vi "Main.vi"() -> ()   [LabVIEW 2013]
panel:
  in  "Continue":bool
  in  "Team Number":string
  in  "Other Name":string
  in  "Name":string(combo)="Other"
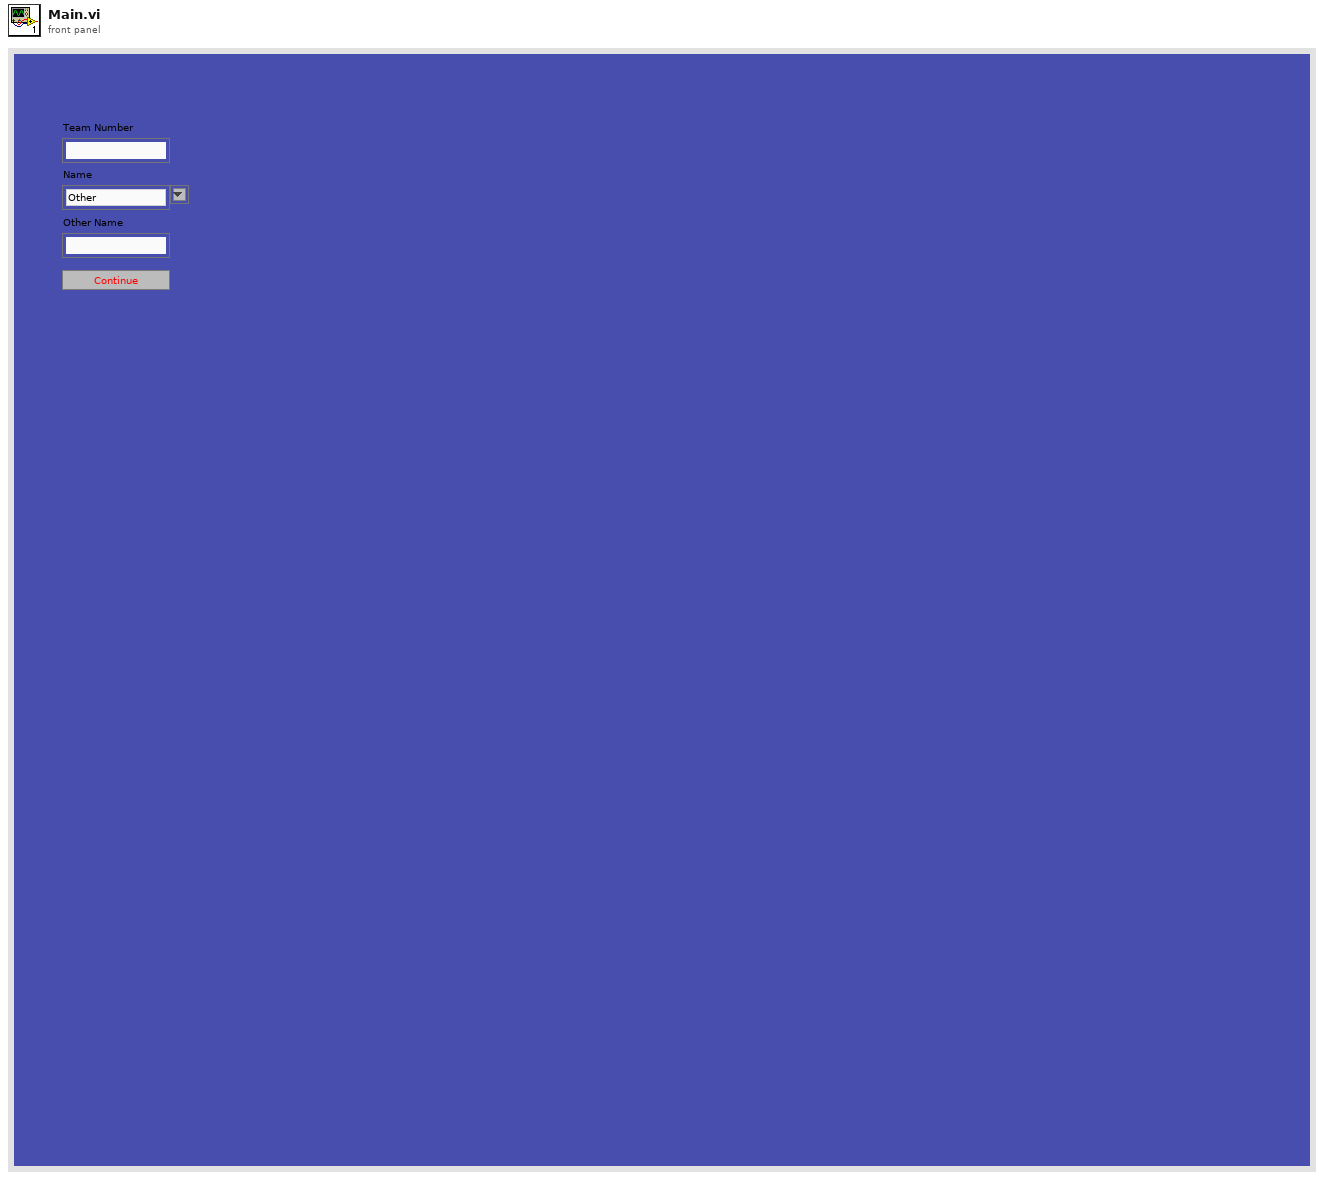
[diagram p1: front panel]
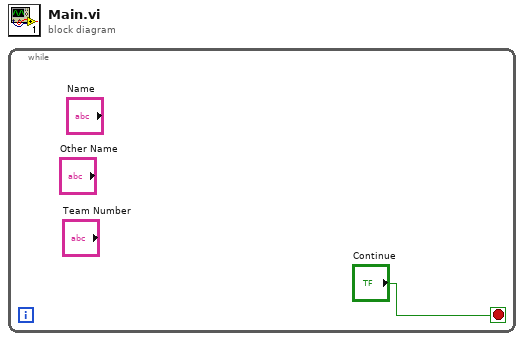
[diagram p0: block diagram]
diagram:
  n1 = while {
    stop <- "Continue" stop-if-true
  }
